vi "arduino sensirion read to stream and log v2 (sub-vi).vi"(0 "logfile refnum":refnum<file>, 1 "VISA resource name (COM3)":refnum<visa-resource-name>="COM3", 2 "stop? tag channel":T1, 3 "abort? (F)":bool, 5 "read byte count (512)":u32=512, 7 "expected num sensors (12)":i32=12, 9 "baud rate (576000)":u32=576000, 11 "error in (no error)":errorcluster) -> (4 "logfile refnum out":refnum<file>, 8 "sensor data cluster\nstream channel":T2, 15 "error out":errorcluster)   [LabVIEW 2021]
uses:
  <extravilib>/ChannelInstances/Stream-t'sensirion_data_with_time.ctl'/)Channel.ctl
  type-defs/sensirion_data_with_time.ctl
  controls/sensirion_flow_sensor_data.ctl
  <extravilib>/ChannelInstances/Tag-bool/))Channel.ctl
  <extravilib>/ChannelInstances/Stream-t'sensirion_data_with_time.ctl'/EndpointRead.vi
  <extravilib>/ChannelInstances/Stream-t'sensirion_data_with_time.ctl'/Endpoint.vi
  <extravilib>/ChannelInstances/Tag-bool/EndpointRead.vi
  <vilib>/Instr/_visa.llb/VISA Configure Serial Port (Instr).vi
  <extravilib>/ChannelInstances/Tag-bool/Instantiate.vi
  <extravilib>/ChannelInstances/Tag-bool/Endpoint.vi
  <extravilib>/ChannelInstances/Stream-t'sensirion_data_with_time.ctl'/Instantiate.vi
  <extravilib>/ChannelInstances/Stream-t'sensirion_data_with_time.ctl'/)Channel.vi
  <resource>/ChannelSupport/_ChannelSupport/WaitIfNeeded.vi
  <extravilib>/ChannelInstances/Stream-t'sensirion_data_with_time.ctl'.lvlib
  <extravilib>/ChannelInstances/Tag-bool.lvlib
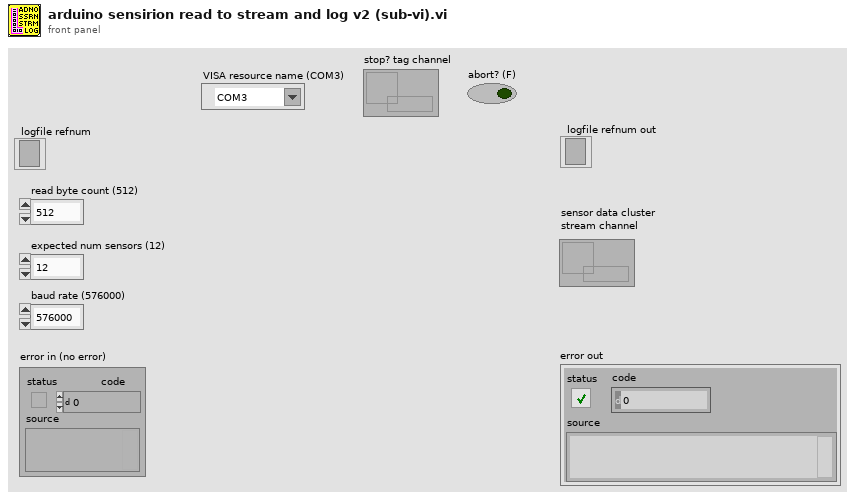
[diagram p1: front panel]
types:
  T1 = typedef "Tag-bool.lvlib/))Channel.ctl" = refnum<queue>
  T2 = typedef "Stream-t'sensirion_data_with_time.ctl'.lvlib/)Channel.ctl" = refnum<queue>
  T3 = typedef "sensirion_data_with_time.ctl" = cluster{"sensor data array":T4[], "relative timestamp":dbl, "error":errorcluster}
  T4 = typedef "sensirion_flow_sensor_data.ctl" = cluster{"flow rate \n":dbl[unit], "flow val. status":bool, "temperature":dbl[unit], "temp. val status":bool, "air in line?":bool, "high flow?":bool, "flag. val status":bool}
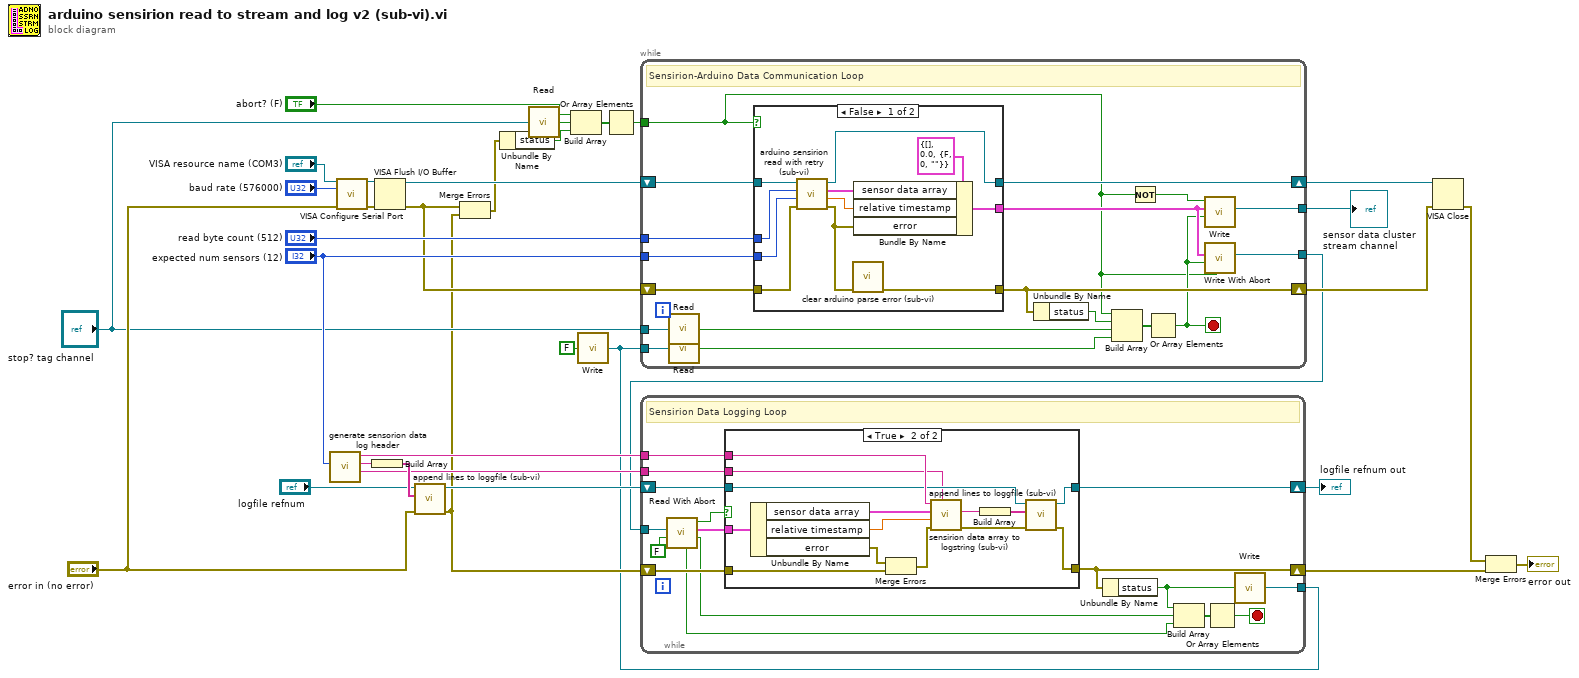
[diagram p0: block diagram]
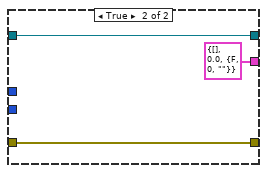
[diagram p2: hidden frame]
diagram:
  n1 = call "generate sensorion data log header.vi"("num sensors"="expected num sensors (12)") -> ("delimiter"=w20:string, "sensor data header string"=w29:string, "value format"=w23:string)  [unwired: 8 in]
  n2 = call-poly "VISA Configure Serial Port"("VISA resource name"="VISA resource name (COM3)", "baud rate (9600)"="baud rate (576000)", "error in (no error)"="error in (no error)") -> ("VISA resource name out"=w31:refnum<visa-resource-name>, "error out"=w30:errorcluster)  [unwired: 11 in]
  n3 = Build Array(w29) -> (w28:string[])
  n4 = VISA Flush I/O Buffer(VISA resource name=w31, error in (no error)=w30) -> (VISA resource name out=w26:refnum<visa-resource-name>, error out=w4:errorcluster)  [unwired: 1 in]
  n5 = call "append lines to loggfile (sub-vi).vi"("error in (no error)"="error in (no error)", "string array"=w28, "file refnum"="logfile refnum") -> ("error out"=w3:errorcluster, "file refnum out"=w22:refnum<file>)  [unwired: 7 in]
  n6 = Merge Errors(w4, w3) -> (w2:errorcluster)
  n7 = Unbundle By Name(w2) -> ("status"=w8:bool)
  n8 = call <extravilib>:"Read.vi"("channel"="stop? tag channel") -> ("element"=w9:bool)  [unwired: 1 in, 1 out]
  n9 = Build Array("abort? (F)", w9, w8) -> (w10:bool[])
  n10 = call <extravilib>:"Write.vi"("element"=FALSE) -> ("channel"=w1:T1)  [unwired: 1 out]
  n11 = Or Array Elements(Boolean array=w10) -> (logical OR=w12:bool)
  n12 = while {
    tunnel: "read byte count (512)" -> [w51]
    tunnel: [w47] -> w14
    tunnel: "expected num sensors (12)" -> [w46]
    shift-right: [w43] -> w19
    shift-left: w4 -> [w49]
    tunnel: [w45] -> w21
    tunnel: "stop? tag channel" -> [w44]
    tunnel: w1 -> [w41]
    tunnel: w12 -> [w35]
    shift-right: [w42] -> w18
    shift-left: w26 -> [w50]
    stop <- w36 stop-if-true
    # "Sensirion-Arduino Data Communication Loop"
    n13 = call <extravilib>:"Read.vi"("channel"=w44) -> ("element"=w39:bool)  [unwired: 1 in, 1 out]
    n14 = call <extravilib>:"Read.vi"("channel"=w41) -> ("element"=w38:bool)  [unwired: 1 in, 1 out]
    n15 = case shown="False" w35 {
      tunnel: w51 -> [w62 _]
      tunnel: w50 -> [w61 w65]
      tunnel: w49 -> [w60 w63]
      tunnel: [w57 T3 {"sensor data array"=[], "relative timestamp"=0.0, "error"={"status"=FALSE, "code"=0, "source"=""}} ("Cluster")] -> w48
      tunnel: w46 -> [w56 _]
      tunnel: [w53 w63] -> w43
      tunnel: [w55 w65] -> w42
      frame False {
        n16 = call "arduino sensirion read with retry (sub-vi).vi"("error in (no error)"=w60, "expected num sensors (12)"=w56, "read byte count (512)"=w62, "VISA resource name"=w61) -> ("error out"=w54:errorcluster, "relative timestamp"=w52:dbl, "sensor data array"=w58:T4[], "VISA resource name out"=w55:refnum<visa-resource-name>)  [unwired: 3 in, 1 out]
        n17 = call "clear arduino parse error (sub-vi).vi"("error in"=w54) -> ("error out"=w53:errorcluster)  [unwired: 10 in]
        n18 = Bundle By Name(cluster=T3 {"sensor data array"=[], "relative timestamp"=0.0, "error"={"status"=FALSE, "code"=0, "source"=""}} ("Cluster"), "sensor data array"=w58, "relative timestamp"=w52, "error"=w54) -> (w57:T3)
      }
      frame True {
      }
    }
    n19 = Unbundle By Name(w43) -> ("status"=w40:bool)
    n20 = Build Array(w35, w40, w39, w38) -> (w37:bool[])
    n21 = Not(x=w35) -> (.not. x?=w34:bool)
    n22 = Or Array Elements(Boolean array=w37) -> (logical OR=w36:bool)
    n23 = call <extravilib>:"Write.vi"("last element? (F)"=w36, "element"=w48, "element valid? (T)"=w34) -> ("channel"=w45:T2)  [unwired: 6 in, 2 out]
    n24 = call <extravilib>:"Write With Abort.vi"("abort"=w35, "last element? (F)"=w36, "element"=w48) -> ("channel"=w47:T2)  [unwired: 5 in, 3 out]
  }
  "sensor data cluster\nstream channel" <- w21
  n25 = while {
    tunnel: w14 -> [w81]
    tunnel: w23 -> [w79]
    shift-right: [w74] -> w15
    shift-left: w3 -> [w76]
    tunnel: w20 -> [w75]
    shift-right: [w77] -> w5
    shift-left: w22 -> [w78]
    tunnel: w1 -> [w66]
    stop <- w68 stop-if-true
    # "Sensirion Data Logging Loop"
    n26 = call <extravilib>:"Read With Abort.vi"("abort"=FALSE, "channel"=w81) -> ("last element?"=w71:bool, "element"=w80:T3, "element valid?"=w73:bool, "aborted?"=w72:bool)  [unwired: 4 in, 2 out]
    n27 = case shown="True" w73 {
      tunnel: w80 -> [_ w97]
      tunnel: w79 -> [_ w96]
      tunnel: w78 -> [w83 w95]
      tunnel: [w83 w90] -> w77
      tunnel: w76 -> [w82 w89]
      tunnel: w75 -> [_ w86]
      tunnel: [w82 w84] -> w74
      frame False {
      }
      frame True {
        n28 = Unbundle By Name(w97) -> ("sensor data array"=w85:T4[], "relative timestamp"=w94:dbl, "error"=w88:errorcluster)
        n29 = Merge Errors(w88, w89) -> (w87:errorcluster)
        n30 = call "sensirion data array to logstring (sub-vi).vi"("delimeter (comma)"=w86, "error in"=w87, "timestamp in relative seconds"=w94, "sensor data array"=w85, "value format (%15s)"=w96) -> ("error out"=w93:errorcluster, "string out"=w91:string)  [unwired: 5 in]
        n31 = Build Array(w91) -> (w92:string[])
        n32 = call "append lines to loggfile (sub-vi).vi"("error in (no error)"=w93, "string array"=w92, "file refnum"=w95) -> ("error out"=w84:errorcluster, "file refnum out"=w90:refnum<file>)  [unwired: 7 in]
      }
    }
    n33 = Unbundle By Name(w74) -> ("status"=w70:bool)
    n34 = Build Array(w70, w71, w72) -> (w69:bool[])
    n35 = Or Array Elements(Boolean array=w69) -> (logical OR=w68:bool)
    n36 = call <extravilib>:"Write.vi"("element"=w70) -> ("channel"=w66:T1)  [unwired: 1 out]
  }
  "logfile refnum out" <- w5
  n37 = VISA Close(VISA resource name=w18, error in (no error)=w19) -> (error out=w16:errorcluster)
  n38 = Merge Errors(w16, w15) -> (→"error out":errorcluster)
